vi "Unpack for gRPC.vi"(8 "error in":errorcluster, 9 "configuration / results":enum16{"Configuration", "Results"}(ring), 10 "any":T1, 11 "measurement customizations in":refnum<class "Measurement Plugin.lvclass">) -> (0 "error out":errorcluster, 2 "data value":variant, 3 "measurement customizations out":refnum<class "Measurement Plugin.lvclass">)   [LabVIEW 2024, in "PMIC_Efficiency_DMM.lvlib" / "Measurement Plugin.lvclass"]
uses:
  Measurement Plugin.lvclass
  <vilib>/gRPC/LabVIEW gRPC Library/Shared/Any.ctl
  C:/Program Files/National Instruments/LabVIEW 2024/vi.lib/MeasurementLink/MeasurementLink Measurement Server/Measurement Plugin Service/Measurement Plugin Service.lvclass
  Measurement Configuration.ctl
  measurementlink-labview-examples-2.0.0.1/NI-DMM Measurement/NIDmmMeasurement/ResolutionInDigits.ctl
  Measurement Results.ctl
  <vilib>/gRPC/Generated APIs/ni/protobuf/types/RPC Messages/ni_protobuf_types_DoubleXYData.ctl
  a521b266-ce99-437c-923d-067dcf1e07fd.vi
  3ecd018e-d556-4cbc-bc60-c4ba57204520.vi
  <vilib>/gRPC/LabVIEW gRPC Library/Server API/Translate Protobuf Error.vi
  <vilib>/AdvancedString/1D String Array to Delimited String.vi
  <vilib>/gRPC/LabVIEW gRPC Library/Server API/Server/Get Server DLL Path.vi
  PMIC_Efficiency_DMM.lvlib
  <vilib>/MeasurementLink/MeasurementLink Measurement Server/Measurement Plugin Service/Measurement Plugin Service.lvclass
  measurementlink-labview-examples-2.0.0.1/NI-DMM Measurement/NIDmmMeasurement/NIDmmMeasurement.lvlib
  <vilib>/gRPC/Generated APIs/ni/protobuf/types/ni.protobuf.types.lvlib
  <vilib>/gRPC/LabVIEW gRPC Library/grpc-lvsupport-release.lvlib
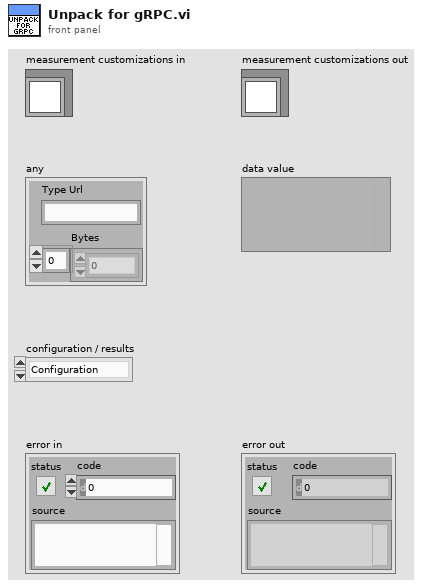
[diagram p1: front panel]
types:
  T1 = typedef "grpc-lvsupport-release.lvlib/Any.ctl" = cluster{"Type Url":string, "Bytes":u8[]}
  T2 = typedef "grpc-lvsupport-release.lvlib/grpcId.ctl" = u64
  T3 = typedef "PMIC_Efficiency_DMM.lvlib/Measurement Configuration.ctl" = cluster{"Vin Pin Name":string, "Source Voltage Level (V)":dbl, "Source Current Limit (A)":dbl, "Eload Pin Name":string, "Load Voltage Limit (V)":dbl, "Points":i32, "Current Load Level Start":dbl, "Current Load Level Stop":dbl, "Vout Pin Name":string, "Range":dbl, "Resolution in Digits":T4}
  T4 = typedef "NIDmmMeasurement.lvlib/ResolutionInDigits.ctl" = enum32{"3 1/2", "4 1/2", "5 1/2", "6 1/2", "7 1/2"}
  T5 = typedef "PMIC_Efficiency_DMM.lvlib/Measurement Results.ctl" = cluster{"Vin":dbl[], "Vout":dbl[], "Iin":dbl[], "Iout":dbl[], "Efficiency":T6}
  T6 = typedef "ni.protobuf.types.lvlib/ni_protobuf_types_DoubleXYData.ctl" = cluster{"x_data":dbl[], "y_data":dbl[]}
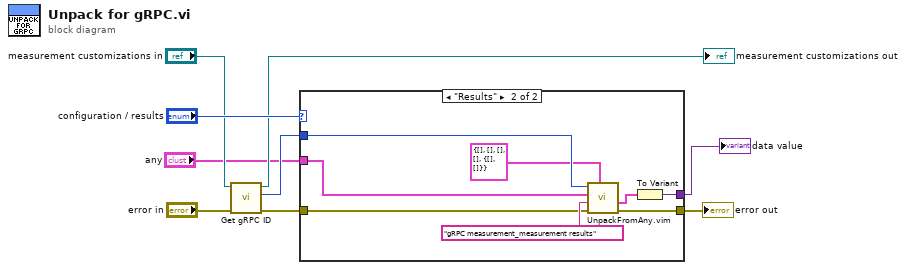
[diagram p0: block diagram]
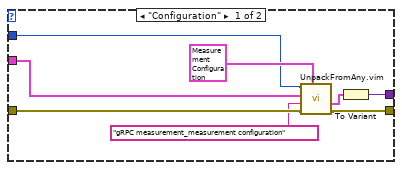
[diagram p2: hidden frame]
diagram:
  n1 = call <vilib>:"Get gRPC ID.vi"("error in"="error in", "measurement plugin service in"="measurement customizations in") -> ("error out"=w6:errorcluster, "gRPC ID"=w3:T2, "measurement plugin service out"=→"measurement customizations out":refnum<class "Measurement Plugin.lvclass">)  [unwired: 7 in]
  n2 = case shown="\"Results\"" "configuration / results" {
    tunnel: w6 -> [w15 w19]
    tunnel: "any" -> [w10 w18]
    tunnel: w3 -> [w12 w22]
    tunnel: [w16 w23] -> w9
    tunnel: [w17 w25] -> w1
    frame "Configuration" {
      n3 = call "UnpackFromAny.vim"("Data Type"=T3 {"Vin Pin Name"="", "Source Voltage Level (V)"=3.0, "Source Current Limit (A)"=1.0, "Eload Pin Name"="", "Load Voltage Limit (V)"=5.0, "Points"=10, "Current Load Level Start"=0.1, "Current Load Level Stop"=1.0, "Vout Pin Name"="", "Range"=10.0, "Resolution in Digits"=enum."5 1/2"} ("Measurement Configuration"), "error in"=w15, "Message Type"="gRPC measurement_measurement configuration", "Any"=w10, "gRPCid in"=w12) -> ("error out"=w16:errorcluster, "Unpacked Value"=w14:T3)  [unwired: 4 in, 1 out]
      n4 = To Variant(anything=w14) -> (Variant=w17:variant)
    }
    frame "Results" {
      n5 = call "UnpackFromAny.vim"("Data Type"=T5 {"Vin"=[], "Vout"=[], "Iin"=[], "Iout"=[], "Efficiency"={"x_data"=[], "y_data"=[]}} ("Measurement Results"), "error in"=w19, "Message Type"="gRPC measurement_measurement results", "Any"=w18, "gRPCid in"=w22) -> ("error out"=w23:errorcluster, "Unpacked Value"=w24:T5)  [unwired: 4 in, 1 out]
      n6 = To Variant(anything=w24) -> (Variant=w25:variant)
    }
  }
  "error out" <- w9
  "data value" <- w1
